vi "raptor_new_scan.vi"(8 "error in (no error)":errorcluster) -> (0 "error out":errorcluster)   [LabVIEW 2016]
doc: "Raptor: Begins a new scan, clearing any existing scan."
uses:
  typedef/raptor_message.ctl
  typedef/raptor_image.ctl
  <vilib>/vision/Image Controls.llb/IMAQ Image.ctl
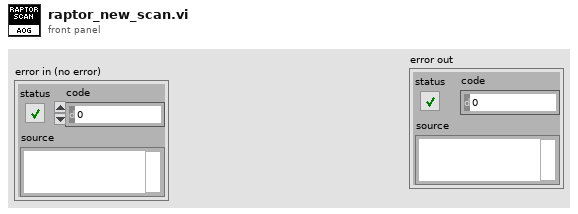
[diagram p1: front panel]
types:
  T1 = typedef "raptor_image.ctl" = cluster{"Data":variant, "Image":T2}
  T2 = typedef "IMAQ Image.ctl" = refnum<image>
  T3 = typedef "raptor_message.ctl" = cluster{"Message":enum16{"start", "stop", "initialise", "shutdown", "end scan", "new scan", "set depth"}, "Data":variant}
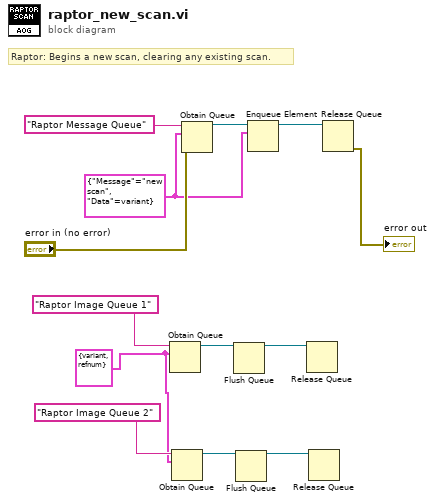
[diagram p0: block diagram]
diagram:
  w1 = T1 {"Data"=variant, "Image"=refnum} ("Cluster")
  w10 = T3 {"Message"=enum."new scan", "Data"=variant} ("Cluster")
  # "Raptor: Begins a new scan, clearing any existing scan."
  n1 = Obtain Queue(name (unnamed)="Raptor Image Queue 1", element data type=w1) -> (queue out=w6:refnum<queue>)  [unwired: 3 in, 2 out]
  n2 = Obtain Queue(name (unnamed)="Raptor Image Queue 2", element data type=w1) -> (queue out=w3:refnum<queue>)  [unwired: 3 in, 2 out]
  n3 = Obtain Queue(name (unnamed)="Raptor Message Queue", element data type=w10, error in (no error)="error in (no error)") -> (queue out=w11:refnum<queue>)  [unwired: 2 in, 2 out]
  n4 = Flush Queue(queue=w6) -> (queue out=w5:refnum<queue>)  [unwired: 1 in, 2 out]
  n5 = Flush Queue(queue=w3) -> (queue out=w4:refnum<queue>)  [unwired: 1 in, 2 out]
  n6 = Enqueue Element(queue=w11, element=w10) -> (queue out=w9:refnum<queue>)  [unwired: 2 in, 2 out]
  n7 = Release Queue(queue=w5) -> ()  [unwired: 2 in, 3 out]
  n8 = Release Queue(queue=w4) -> ()  [unwired: 2 in, 3 out]
  n9 = Release Queue(queue=w9) -> (error out=→"error out":errorcluster)  [unwired: 2 in, 2 out]
